vi "Complex Matrix.vi"() -> (0 "error out":errorcluster, 3 "Passed?":bool)   [LabVIEW 2009]
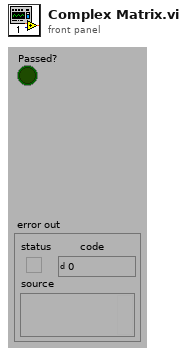
[diagram p1: front panel]
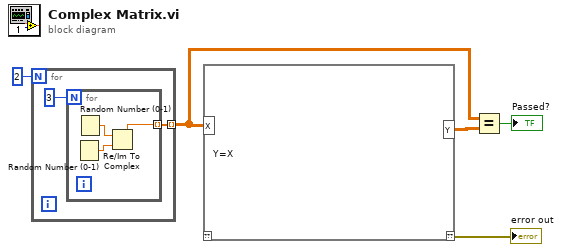
[diagram p0: block diagram]
diagram:
  n1 = for {
    N: 2 -> [_]
    tunnel: [w6] -> w3 mode=indexing
    n2 = for {
      N: 3 -> [_]
      tunnel: [w8] -> w6 mode=indexing
      n3 = Random Number (0-1)() -> (number: 0 to 1=w10:dbl)
      n4 = Random Number (0-1)() -> (number: 0 to 1=w9:dbl)
      n5 = Re/Im To Complex(1:w10, 2:w9) -> (0:w8:cdb)
    }
  }
  n6 = script code="Y=X"("X"=w3) -> ("??"=→"error out":errorcluster, "Y"=w2:cdb[][])  [unwired: 1 in]
  n7 = Equal?(x=w3, y=w2) -> (x = y?=→"Passed?":bool)
